vi "setGlobals5.vi"() -> ()   [LabVIEW 2011]
uses:
  globals.vi
panel:
  in  "Tab Control":T1(tab)
  in  "Multiprogrammer Card Slots":T2={"Relay Card Slots"={"Card 1"=10, "Card 2"=11, "Card 3"=12, "Card 4"=13, "Card 5"=14}, "Quad D/A Card Slots"={"Card 1"=4, "Card 2"=5, "Card 3"=7, "Card 4"=8, "Card 5"=9, "Card 6 (12-bit)"=9}, "A/D Card Slots"={"Scanner"=0, "High-Speed A/D"=1, "Timer"=2}} {"A/D Card Slots"."Timer" items=["400@", "401A", "402B", "403C", "404D", "405E", "406F", "407G", "408H", "409I", "410J", "411K", "412L", "413M", "414N"]; "A/D Card Slots"."High-Speed A/D" items=["400@", "401A", "402B", "403C", "404D", "405E", "406F", "407G", "408H", "409I", "410J", "411K", "412L", "413M", "414N"]; "A/D Card Slots"."Scanner" items=["400@", "401A", "402B", "403C", "404D", "405E", "406F", "407G", "408H", "409I", "410J", "411K", "412L", "413M", "414N"]; "Quad D/A Card Slots"."Card 6 (12-bit)" items=["400@", "401A", "402B", "403C", "404D", "405E", "406F", "407G", "408H", "409I", "410J", "411K", "412L", "413M", "414N"]; "Quad D/A Card Slots"."Card 1" items=["400@", "401A", "402B", "403C", "404D", "405E", "406F", "407G", "408H", "409I", "410J", "411K", "412L", "413M", "414N"]; "Quad D/A Card Slots"."Card 2" items=["400@", "401A", "402B", "403C", "404D", "405E", "406F", "407G", "408H", "409I", "410J", "411K", "412L", "413M", "414N"]; "Quad D/A Card Slots"."Card 3" items=["400@", "401A", "402B", "403C", "404D", "405E", "406F", "407G", "408H", "409I", "410J", "411K", "412L", "413M", "414N"]; "Quad D/A Card Slots"."Card 4" items=["400@", "401A", "402B", "403C", "404D", "405E", "406F", "407G", "408H", "409I", "410J", "411K", "412L", "413M", "414N"]; "Quad D/A Card Slots"."Card 5" items=["400@", "401A", "402B", "403C", "404D", "405E", "406F", "407G", "408H", "409I", "410J", "411K", "412L", "413M", "414N"]; "Relay Card Slots"."Card 5" items=["400@", "401A", "402B", "403C", "404D", "405E", "406F", "407G", "408H", "409I", "410J", "411K", "412L", "413M", "414N"]; "Relay Card Slots"."Card 4" items=["400@", "401A", "402B", "403C", "404D", "405E", "406F", "407G", "408H", "409I", "410J", "411K", "412L", "413M", "414N"]; "Relay Card Slots"."Card 3" items=["400@", "401A", "402B", "403C", "404D", "405E", "406F", "407G", "408H", "409I", "410J", "411K", "412L", "413M", "414N"]; "Relay Card Slots"."Card 2" items=["400@", "401A", "402B", "403C", "404D", "405E", "406F", "407G", "408H", "409I", "410J", "411K", "412L", "413M", "414N"]; "Relay Card Slots"."Card 1" items=["400@", "401A", "402B", "403C", "404D", "405E", "406F", "407G", "408H", "409I", "410J", "411K", "412L", "413M", "414N"]}
  in  "Mass flow controllers":cluster{"MFC Range":u16, "MFC Name":string}[](array[cluster]) {"MFC Range" items=["0-10 sccm", "0-100 sccm", "0-1000 sccm"]}
  in  "D/A Cards":T3 {"Single-channel D/A (12-bit) Cards"."Channel 1" items=["N2 flow (NMFC1)", "H2 flow (HMFC1)", "Al2 flow (ALMFC1)", "Ga flow 1 (GAMFC1)", "Ga flow 2 (GAMFC2)", "Ga flow 3 (GAMFC3)", "In flow (INMFC1)", "P bubbler (PLMFC1)", "Plasma feed (ASLMFC1)", "P gas (PGMFC1)", "As gas (ASGMFC1)", "p-dopant flow 1 (PDOPMFC1)", "p-dopant flow 2 (PDOPMFC2)", "p-dopant flow 3 (PDOPMFC3)", "n-dopant flow 1 (NDOPMFC1)", "n-dopant flow 2 (NDOPMFC2)", "n-dopant flow 3 (PDOPMFC3)", "bad", "Fe flow 1 (FEMFC1)", "Fe flow 2 (FEMFC2)", "Fe flow 3 (FEMFC3)"]; "Quad D/A (10-bit) Cards"."Channel 4" items=["N2 flow (NMFC1)", "H2 flow (HMFC1)", "Al2 flow (ALMFC1)", "Ga flow 1 (GAMFC1)", "Ga flow 2 (GAMFC2)", "Ga flow 3 (GAMFC3)", "In flow (INMFC1)", "P bubbler (PLMFC1)", "Plasma feed (ASLMFC1)", "P gas (PGMFC1)", "As gas (ASGMFC1)", "p-dopant flow 1 (PDOPMFC1)", "p-dopant flow 2 (PDOPMFC2)", "p-dopant flow 3 (PDOPMFC3)", "n-dopant flow 1 (NDOPMFC1)", "n-dopant flow 2 (NDOPMFC2)", "n-dopant flow 3 (PDOPMFC3)", "bad", "Fe flow 1 (FEMFC1)", "Fe flow 2 (FEMFC2)", "Fe flow 3 (FEMFC3)"]; "Quad D/A (10-bit) Cards"."Channel 3" items=["N2 flow (NMFC1)", "H2 flow (HMFC1)", "Al2 flow (ALMFC1)", "Ga flow 1 (GAMFC1)", "Ga flow 2 (GAMFC2)", "Ga flow 3 (GAMFC3)", "In flow (INMFC1)", "P bubbler (PLMFC1)", "Plasma feed (ASLMFC1)", "P gas (PGMFC1)", "As gas (ASGMFC1)", "p-dopant flow 1 (PDOPMFC1)", "p-dopant flow 2 (PDOPMFC2)", "p-dopant flow 3 (PDOPMFC3)", "n-dopant flow 1 (NDOPMFC1)", "n-dopant flow 2 (NDOPMFC2)", "n-dopant flow 3 (PDOPMFC3)", "bad", "Fe flow 1 (FEMFC1)", "Fe flow 2 (FEMFC2)", "Fe flow 3 (FEMFC3)"]; "Quad D/A (10-bit) Cards"."Channel 2" items=["N2 flow (NMFC1)", "H2 flow (HMFC1)", "Al2 flow (ALMFC1)", "Ga flow 1 (GAMFC1)", "Ga flow 2 (GAMFC2)", "Ga flow 3 (GAMFC3)", "In flow (INMFC1)", "P bubbler (PLMFC1)", "Plasma feed (ASLMFC1)", "P gas (PGMFC1)", "As gas (ASGMFC1)", "p-dopant flow 1 (PDOPMFC1)", "p-dopant flow 2 (PDOPMFC2)", "p-dopant flow 3 (PDOPMFC3)", "n-dopant flow 1 (NDOPMFC1)", "n-dopant flow 2 (NDOPMFC2)", "n-dopant flow 3 (PDOPMFC3)", "bad", "Fe flow 1 (FEMFC1)", "Fe flow 2 (FEMFC2)", "Fe flow 3 (FEMFC3)"]; "Quad D/A (10-bit) Cards"."Channel 1" items=["N2 flow (NMFC1)", "H2 flow (HMFC1)", "Al2 flow (ALMFC1)", "Ga flow 1 (GAMFC1)", "Ga flow 2 (GAMFC2)", "Ga flow 3 (GAMFC3)", "In flow (INMFC1)", "P bubbler (PLMFC1)", "Plasma feed (ASLMFC1)", "P gas (PGMFC1)", "As gas (ASGMFC1)", "p-dopant flow 1 (PDOPMFC1)", "p-dopant flow 2 (PDOPMFC2)", "p-dopant flow 3 (PDOPMFC3)", "n-dopant flow 1 (NDOPMFC1)", "n-dopant flow 2 (NDOPMFC2)", "n-dopant flow 3 (PDOPMFC3)", "bad", "Fe flow 1 (FEMFC1)", "Fe flow 2 (FEMFC2)", "Fe flow 3 (FEMFC3)"]}
  in  "Functions":T4(array[cluster])
  out "output array":string[](array[string])
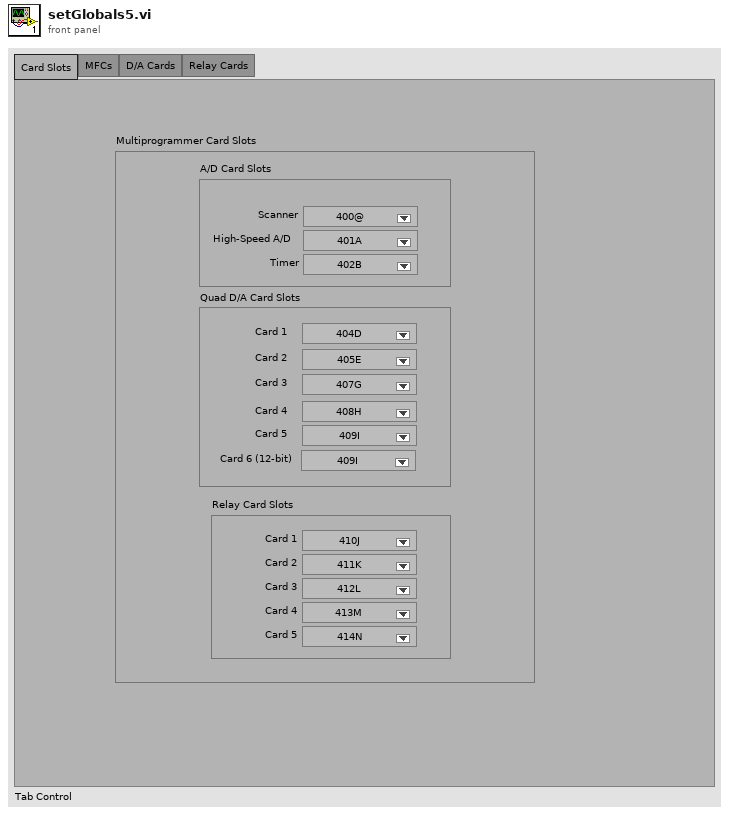
[diagram p1: front panel]
types:
  T1 = enum32{"Card Slots", "MFCs", "D/A Cards", "Relay Cards"}
  T2 = cluster{"Relay Card Slots":cluster{"Card 1":u16, "Card 2":u16, "Card 3":u16, "Card 4":u16, "Card 5":u16}, "Quad D/A Card Slots":cluster{"Card 1":u16, "Card 2":u16, "Card 3":u16, "Card 4":u16, "Card 5":u16, "Card 6 (12-bit)":u16}, "A/D Card Slots":cluster{"Scanner":u16, "High-Speed A/D":u16, "Timer":u16}}
  T3 = cluster{"Quad D/A (10-bit) Cards":cluster{"Channel 1":u16, "Channel 2":u16, "Channel 3":u16, "Channel 4":u16, "Name":string}[], "Single-channel D/A (12-bit) Cards":cluster{"Name":string, "Channel 1":u16}[]}
  T4 = cluster{"Function Group":void[], "Group Name":string, "Function":string}[]
  T5 = cluster{"Channel 1":u16, "Channel 2":u16, "Channel 3":u16, "Channel 4":u16, "Name":string}[]
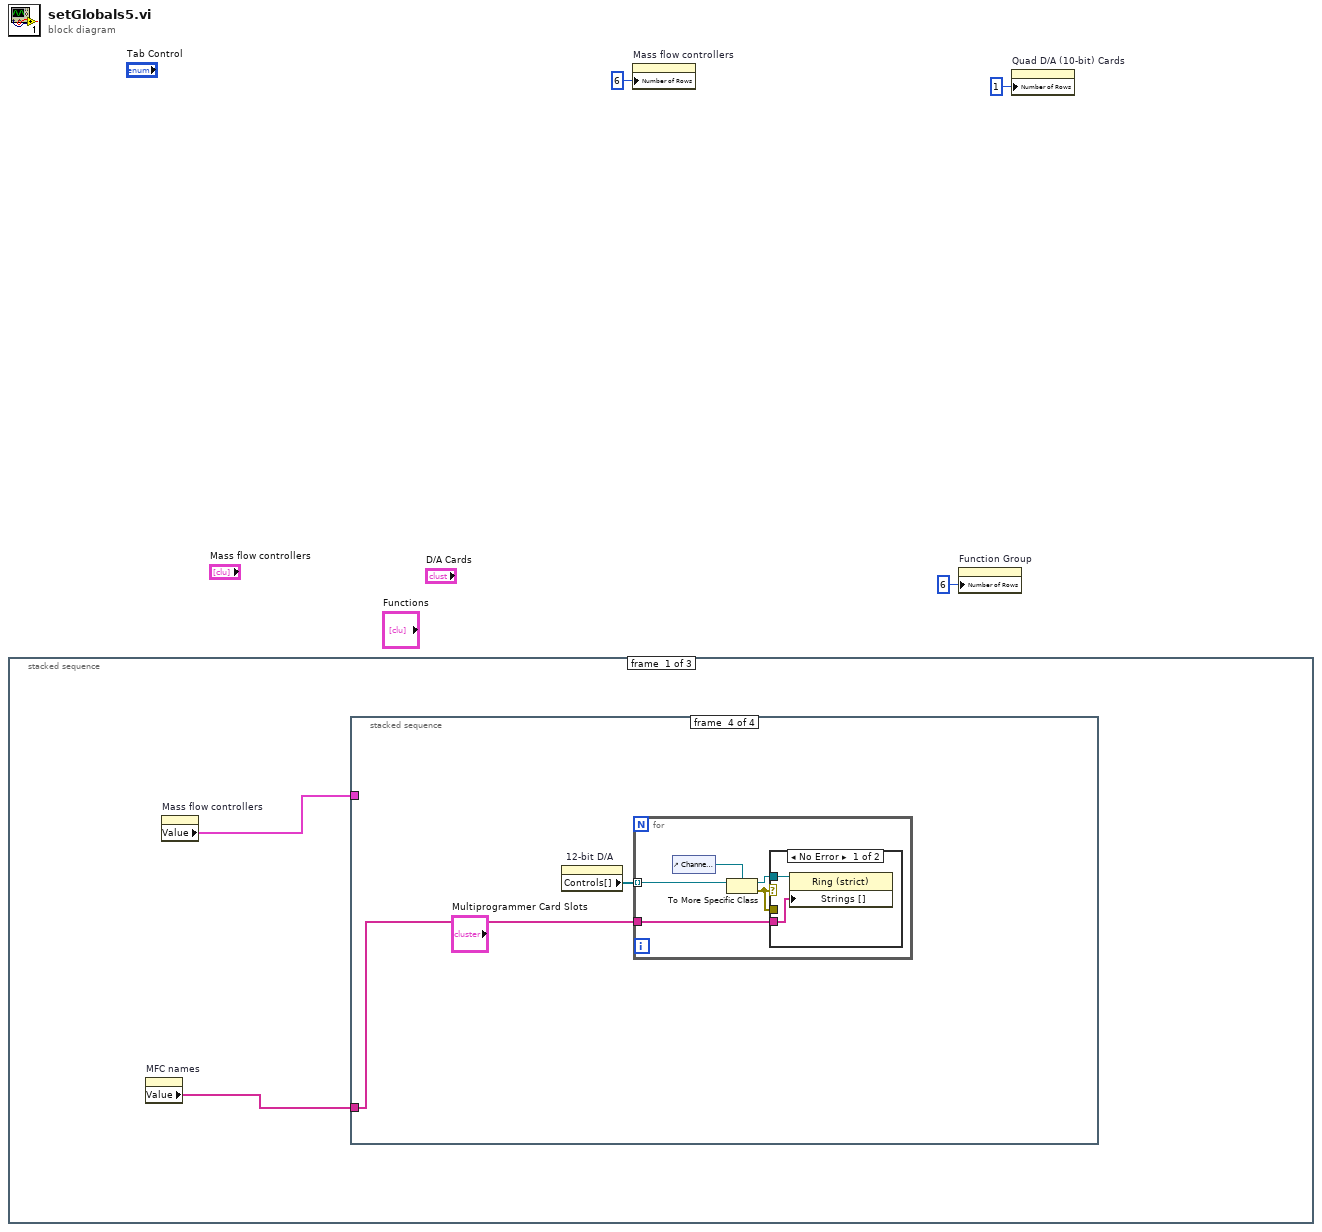
[diagram p0: block diagram]
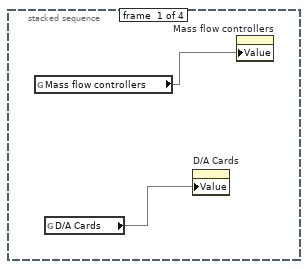
[diagram p2: hidden frame]
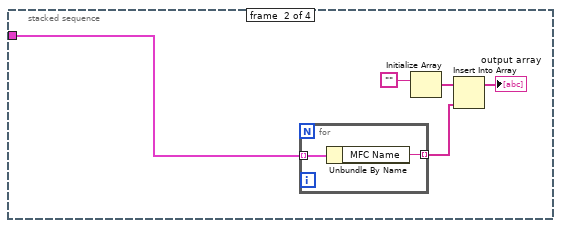
[diagram p3: hidden frame]
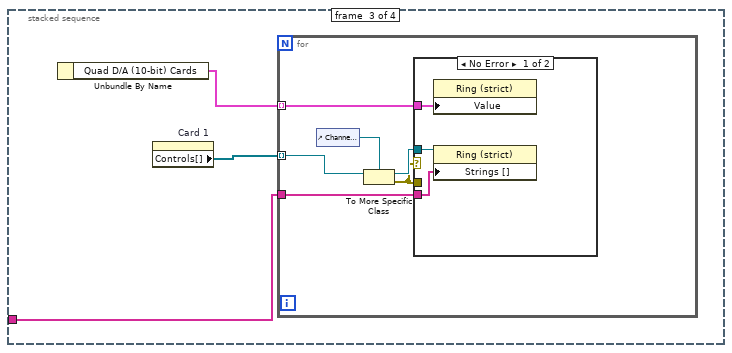
[diagram p4: hidden frame]
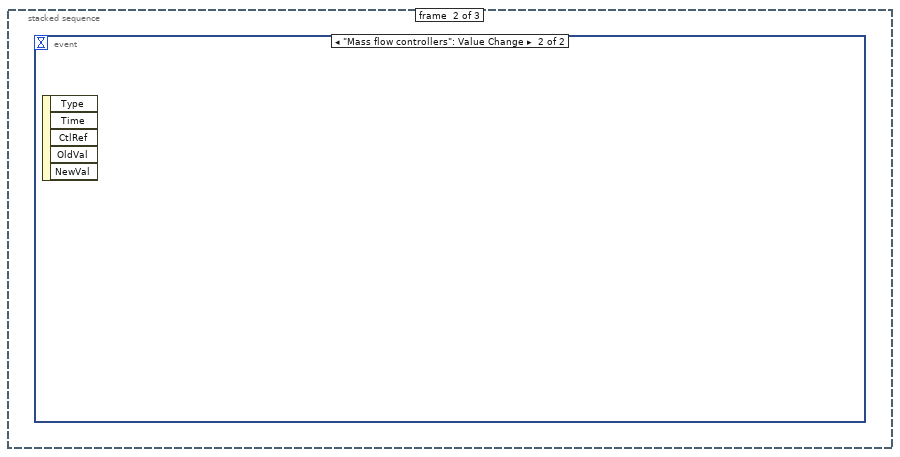
[diagram p7: hidden frame]
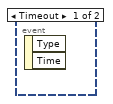
[diagram p8: hidden frame]
diagram:
  n1 = stacked-sequence {
    frame #0 {
      n2 = property on="MFC names" class="Arr (strict)"() -> ("Value"=w5:string[])  [unwired: 2 in, 2 out]
      n3 = property on="Mass flow controllers" class="Arr (strict)"() -> ("Value"=w4:cluster{"MFC Range":u16, "MFC Name":string}[])  [unwired: 2 in, 2 out]
      n4 = stacked-sequence {
        tunnel: w4 -> [_ w9 _ _]
        tunnel: w5 -> [_ _ w16 w27]
        frame #0 {
          n5 = global read "globals.vi" "Mass flow controllers"() -> (w6)
          n6 = global read "globals.vi" "D/A Cards"() -> (w7)
          n7 = property on="D/A Cards" class="Clust (strict)"("Value"=w7) -> ()  [unwired: 2 in, 2 out]
          n8 = property on="Mass flow controllers" class="Arr (strict)"("Value"=w6) -> ()  [unwired: 2 in, 2 out]
        }
        frame #1 {
          n9 = for {
            tunnel: w9 -> [w14] mode=indexing
            tunnel: [w13] -> w11 mode=indexing
            n10 = Unbundle By Name(w14) -> ("MFC Name"=w13:string)
          }
          n11 = Initialize Array("") -> (w10:string[])  [unwired: 1 in]
          n12 = Insert Into Array(array=w10, new element=w11) -> (→"output array":string[])  [unwired: 1 in]
        }
        frame #2 {
          n13 = Unbundle By Name() -> ("Quad D/A (10-bit) Cards"=w15:T5)  [unwired: 1 in]
          n14 = property on="Card 1" class="Clust (strict)"() -> ("Controls[]"=w17:refnum<vi>[])  [unwired: 2 in, 2 out]
          n15 = for {
            tunnel: w17 -> [w20] mode=indexing
            tunnel: w16 -> [w23]
            tunnel: w15 -> [w18] mode=indexing
            n16 = control-ref of="Channel 1"() -> (w19:refnum<vi>)
            n17 = To More Specific Class(target class=w19, reference=w20) -> (specific class reference=w22:refnum<vi>, error out=w21:errorcluster)  [unwired: 1 in]
            n18 = case shown="No Error" w21 {
              tunnel: w22 -> [w26 _]
              tunnel: w21 -> [_ _]
              tunnel: w23 -> [w25 _]
              tunnel: w18 -> [w24 _]
              frame No Error {
                n19 = property class="Ring (strict)"("Value"=w24) -> ()  [unwired: 2 in, 2 out]
                n20 = property class="Ring (strict)"(reference=w26, "Strings []"=w25) -> ()  [unwired: 1 in, 2 out]
              }
              frame Error {
              }
            }
          }
        }
        frame #3 {
          n21 = property on="12-bit D/A" class="Clust (strict)"() -> ("Controls[]"=w28:refnum<vi>[])  [unwired: 2 in, 2 out]
          n22 = for {
            tunnel: w28 -> [w30] mode=indexing
            tunnel: w27 -> [w33]
            n23 = control-ref of="Channel 1"() -> (w29:refnum<vi>)
            n24 = To More Specific Class(target class=w29, reference=w30) -> (specific class reference=w32:refnum<vi>, error out=w31:errorcluster)  [unwired: 1 in]
            n25 = case shown="No Error" w31 {
              tunnel: w32 -> [w34 _]
              tunnel: w31 -> [_ _]
              tunnel: w33 -> [w35 _]
              frame No Error {
                n26 = property class="Ring (strict)"(reference=w34, "Strings []"=w35) -> ()  [unwired: 1 in, 2 out]
              }
              frame Error {
              }
            }
          }
        }
      }
    }
    frame #1 {
      n27 = event shown="[1] \"Mass flow controllers\": Value Change" {
        selector: _ -> [_ _]
        dyn-events: _ -> [_ _]
        timeout: _ -> [_ _]
        event Timeout {
          n28 = event-data() -> ()  [unwired: 1 in, 2 out]
        }
        event "Mass flow controllers": Value Change {
          n29 = event-data() -> ()  [unwired: 1 in, 5 out]
        }
      }
    }
    frame #2 {
    }
  }
  n30 = property on="Mass flow controllers" class="Arr (strict)"("Number of Rows"=u32 6) -> ()  [unwired: 2 in, 2 out]
  n31 = property on="Function Group" class="Arr"("Number of Rows"=u32 6) -> ()  [unwired: 2 in, 2 out]
  n32 = property on="Quad D/A (10-bit) Cards" class="Arr (strict)"("Number of Rows"=u32 1) -> ()  [unwired: 2 in, 2 out]
